vi "Generate_WayPoints_Hopping_LineScan_NOLIGHT.vi"(11 "Input Cluster":T2={"Scan Rate (um/s)"=15.0, "X Start"=15.0, "X End"=15.0, "Y Start"=15.0, "Num_Lines"=15.0, " Z Start"=15.0, "HoppingDistance"=1.0, "V"=15.0, "Z End"=15.0, "Approach Rate Hopping (um/s)"=15.0, "Retract Rate (um/s)"=15.0, "V 2"=15.0, "Approach Rate (um/s)"=15.0}) -> (0 "output cluster":T1)   [LabVIEW 2023]
uses:
  TypeDefs/WayPointCluster.ctl
  User_Vi/Settings.vi
panel:
  out "Numeric":i32
  in  "WayPointCluster":T1
  out "CurrentLine":dbl
  out "X  P":dbl
  out "HoppingDistanceX":dbl
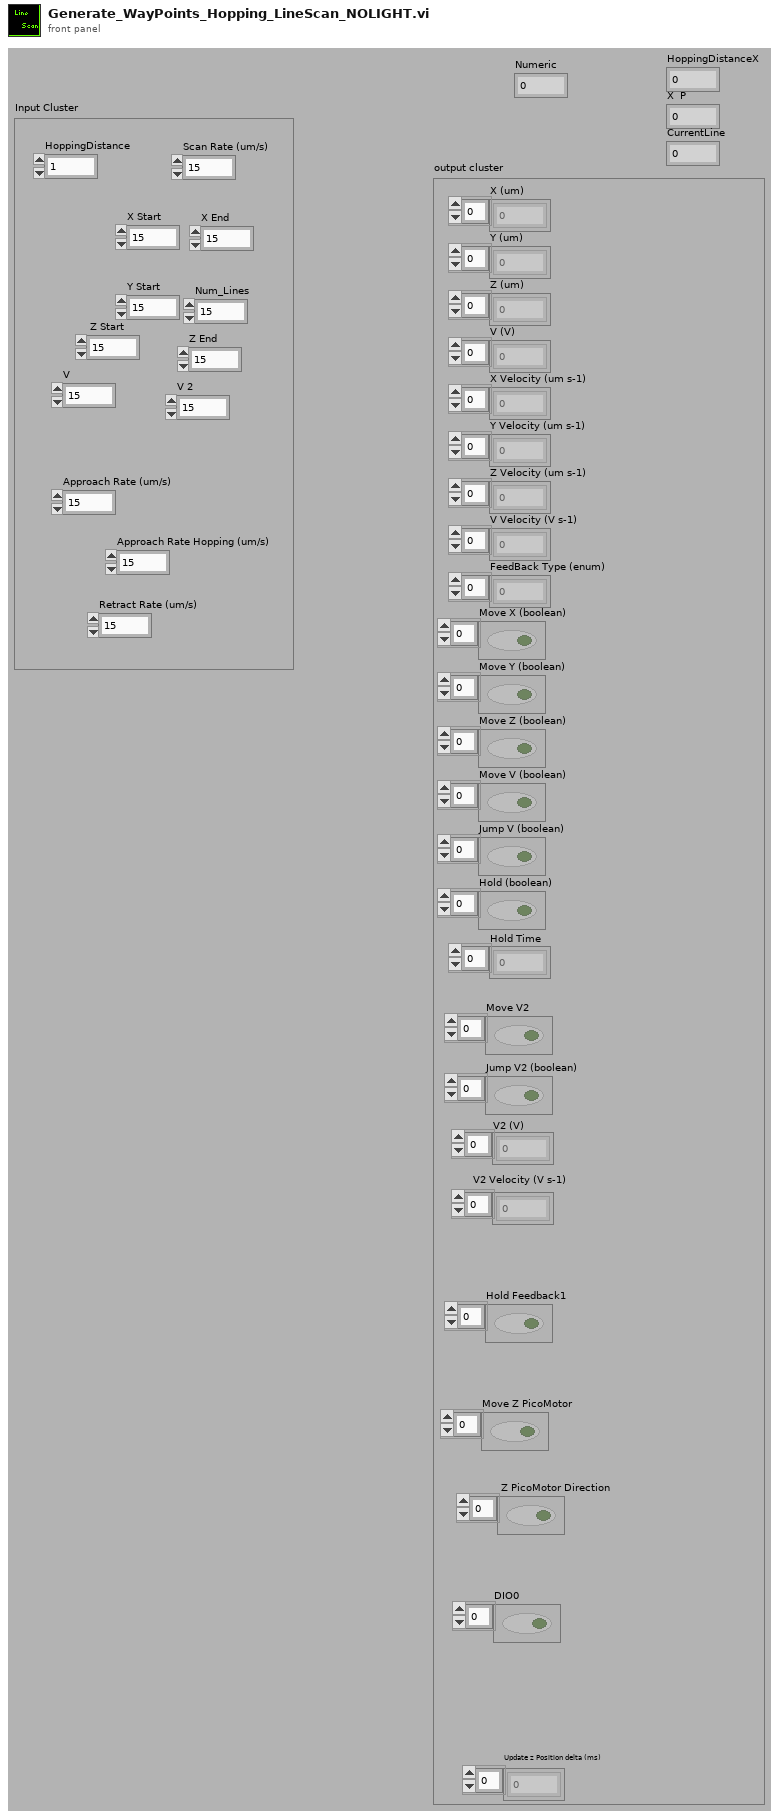
[diagram p1: front panel]
types:
  T1 = typedef "WayPointCluster.ctl" = cluster{"X (um)":dbl[], "Y (um)":dbl[], "Z (um)":dbl[], "V (V)":dbl[], "X Velocity (um s-1)":dbl[], "Y Velocity (um s-1)":dbl[], "Z Velocity (um s-1)":dbl[], "V Velocity (V s-1)":dbl[], "FeedBack Type (enum)":u16[], "Move X (boolean)":bool[], "Move Y (boolean)":bool[], "Move Z (boolean)":bool[], "Move V (boolean)":bool[], "Jump V (boolean)":bool[], "Hold (boolean)":bool[], "Hold Time":u32[], "V2 (V)":dbl[], "Move V2":bool[], "V2 Velocity (V s-1)":dbl[], "Jump V2 (boolean)":bool[], "Update z Position delta (ms)":i16[], "Hold Feedback1":bool[], "Move Z PicoMotor":bool[], " Z PicoMotor Direction":bool[], "DIO0":bool[]}
  T2 = cluster{"Scan Rate (um/s)":dbl, "X Start":dbl, "X End":dbl, "Y Start":dbl, "Num_Lines":dbl, " Z Start":dbl, "HoppingDistance":dbl, "V":dbl, "Z End":dbl, "Approach Rate Hopping (um/s)":dbl, "Retract Rate (um/s)":dbl, "V 2":dbl, "Approach Rate (um/s)":dbl}
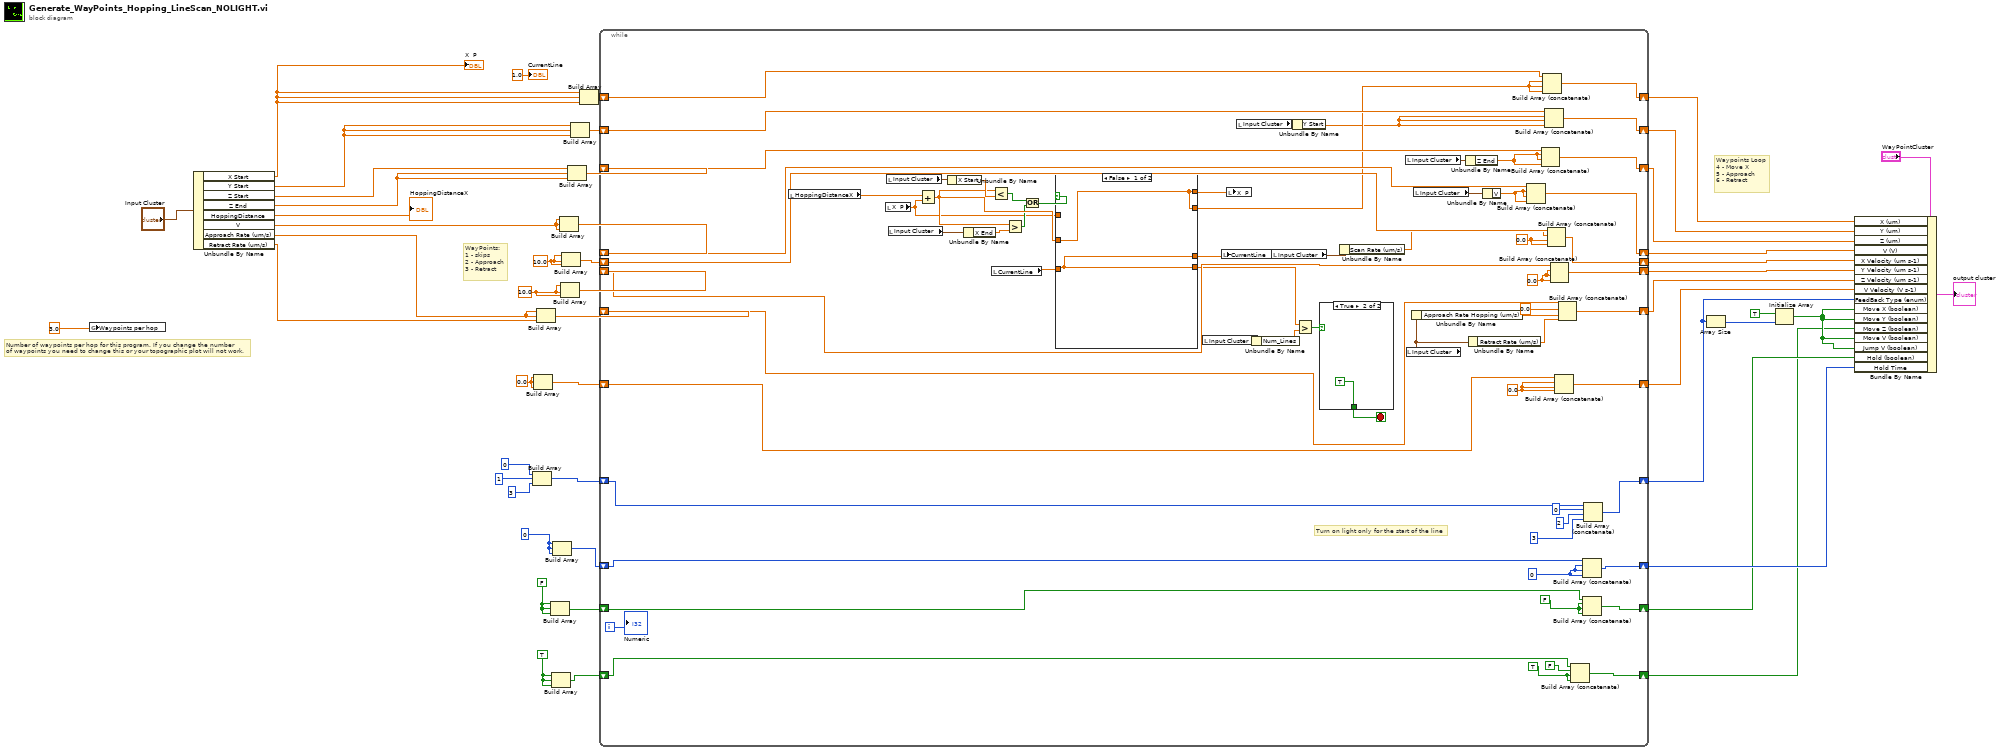
[diagram p0: block diagram]
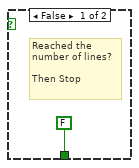
[diagram p2: hidden frame]
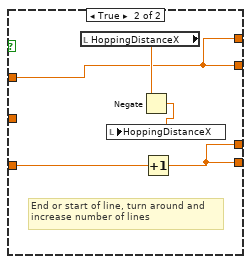
[diagram p3: hidden frame]
diagram:
  w14 = TRUE
  w15 = FALSE
  w23 = u16 0 ("element")
  w9 = 10.0 ("element")
  w10 = 10.0 ("element")
  w12 = 0.0 ("element")
  # "Number of waypoints per hop for this program. If you change the number\nof waypoints you need to change this or your topographic plot will not work."
  # "Waypoints Loop\n4 - Move X\n5 - Approach\n6 - Retract"
  # "WayPoints:\n1 - skips\n2 - Approach\n3 - Retract"
  n1 = global write "Settings.vi" "Waypoints per hop"(3.0) -> ()
  n2 = Unbundle By Name("Input Cluster") -> ("X Start"=w6:dbl, "Y Start"=w5:dbl, "Z Start"=w30:dbl, "Z End"=w7:dbl, "HoppingDistance"=→"HoppingDistanceX":dbl, "V"=w8:dbl, "Approach Rate (um/s)"=w27:dbl, "Retract Rate (um/s)"=w11:dbl)
  "X  P" <- w6
  n3 = Build Array(u16 0 ("element"), u16 1 ("element"), u16 3 ("element")) -> (w33:u16[])
  n4 = Build Array(w12, w12, w12) -> (w24:dbl[])
  n5 = Build Array(w27, w27, w11) -> (w36:dbl[])
  n6 = Build Array(w15, w15, w15) -> (w19:bool[])
  n7 = Build Array(w14, w14, w14) -> (w17:bool[])
  n8 = Build Array(w23, w23, w23) -> (w22:u16[])
  n9 = Build Array(w8, w8, w8) -> (w41:dbl[])
  n10 = Build Array(w10, w10, w10) -> (w38:dbl[])
  n11 = Build Array(w9, w9, w9) -> (w39:dbl[])
  n12 = Build Array(w30, w7, w7) -> (w43:dbl[])
  n13 = Build Array(w5, w5, w5) -> (w44:dbl[])
  n14 = Build Array(w6, w6, w6) -> (w46:dbl[])
  n15 = while {
    shift-right: [w112] -> w45
    shift-left: w46 -> [w113]
    shift-right: [w104] -> w31
    shift-left: w44 -> [w95]
    shift-right: [w103] -> w42
    shift-left: w43 -> [w111]
    shift-right: [w102] -> w40
    shift-left: w41 -> [w110]
    shift-right: [w101] -> w3
    shift-left: w39 -> [w109]
    shift-right: [w77] -> w37
    shift-left: w38 -> [w108]
    shift-right: [w100] -> w35
    shift-left: w36 -> [w107]
    shift-right: [w99] -> w34
    shift-left: w24 -> [w106]
    shift-right: [w98] -> w29
    shift-left: w33 -> [w105]
    shift-right: [w71] -> w21
    shift-left: w22 -> [w72]
    shift-right: [w70] -> w20
    shift-left: w19 -> [w68]
    shift-right: [w65] -> w16
    shift-left: w17 -> [w64]
    i -> [w67]
    stop <- w85 stop-if-true
    w66 = TRUE
    w69 = FALSE
    w62 = u16 0 ("element")
    w59 = 0.0 ("element")
    w58 = 0.0 ("element")
    w61 = 0.0 ("element")
    # "Turn on light only for the start of the line"
    n16 = local read "HoppingDistanceX"() -> (w78:dbl)
    n17 = local read "X  P"() -> (w79:dbl)
    n18 = local read "Input Cluster"() -> (w115:T2)
    n19 = local read "Input Cluster"() -> (w114:T2)
    n20 = Add(x=w78, y=w79) -> (x+y=w91:dbl)
    n21 = Unbundle By Name(w115) -> ("X Start"=w94:dbl)
    n22 = Unbundle By Name(w114) -> ("X End"=w92:dbl)
    n23 = local read "CurrentLine"() -> (w55:dbl)
    n24 = Less?(x=w91, y=w94) -> (x < y?=w93:bool)
    n25 = Greater?(x=w91, y=w92) -> (0:w90:bool)
    n26 = Or(x=w93, y=w90) -> (x .or. y?=w89:bool)
    n27 = case shown="False" w89 {
      tunnel: w91 -> [w119 _]
      tunnel: [w119 w122] -> w56
      tunnel: w79 -> [_ w122]
      tunnel: [w118 w121] -> w84
      tunnel: [w118 w121] -> w83
      tunnel: [w119 w122] -> w63
      tunnel: w55 -> [w118 w120]
      frame False {
      }
      frame True {
        # "End or start of line, turn around and \nincrease number of lines"
        n28 = local read "HoppingDistanceX"() -> (w124:dbl)
        n29 = Negate(x=w124) -> (-x=w123:dbl)
        n30 = local write "HoppingDistanceX"(w123) -> ()
        n31 = Increment(x=w120) -> (x+1=w121:dbl)
      }
    }
    n32 = local read "Input Cluster"() -> (w88:T2)
    n33 = local write "CurrentLine"(w83) -> ()
    n34 = local write "X  P"(w63) -> ()
    n35 = local read "Input Cluster"() -> (w73:T2)
    n36 = Unbundle By Name(w88) -> ("Num_Lines"=w87:dbl)
    n37 = local read "Input Cluster"() -> (w52:T2)
    n38 = Unbundle By Name(w73) -> ("Y Start"=w50:dbl)
    n39 = Greater?(x=w84, y=w87) -> (0:w86:bool)
    n40 = case shown="True" w86 {
      tunnel: [FALSE TRUE] -> w85
      frame False {
        # "Reached the \nnumber of lines?\n\nThen Stop"
      }
      frame True {
      }
    }
    n41 = Unbundle By Name(w52) -> ("Scan Rate (um/s)"=w51:dbl)
    n42 = local read "Input Cluster"() -> (w97:T2)
    n43 = local read "Input Cluster"() -> (w76:T2)
    n44 = Unbundle By Name(w76) -> ("Approach Rate Hopping (um/s)"=w80:dbl)
    n45 = local read "Input Cluster"() -> (w96:T2)
    n46 = Unbundle By Name(w97) -> ("Z End"=w54:dbl)
    n47 = Unbundle By Name(w76) -> ("Retract Rate (um/s)"=w74:dbl)
    n48 = Unbundle By Name(w96) -> ("V"=w57:dbl)
    n49 = Build Array (concatenate)(w110, w57, w57, w57) -> (w102:dbl[])
    n50 = Build Array (concatenate)(w111, w54, w54, w54) -> (w103:dbl[])
    n51 = Build Array (concatenate)(w113, w56, w56, w56) -> (w112:dbl[])
    n52 = Build Array (concatenate)(w95, w50, w50, w50) -> (w104:dbl[])
    n53 = Build Array (concatenate)(w109, w51, w58, w58) -> (w101:dbl[])
    n54 = Build Array (concatenate)(w108, w59, w59, w59) -> (w77:dbl[])
    n55 = Build Array (concatenate)(w106, w61, w61, w61) -> (w99:dbl[])
    n56 = Build Array (concatenate)(w107, 0.0 ("element"), w80, w74) -> (w100:dbl[])
    n57 = Build Array (concatenate)(w64, FALSE, w66, w66) -> (w65:bool[])
    n58 = Build Array (concatenate)(w72, w62, w62, w62) -> (w71:u16[])
    n59 = Build Array (concatenate)(w68, w69, w69, w69) -> (w70:bool[])
    n60 = Build Array (concatenate)(w105, u16 0 ("element"), u16 2 ("element"), u16 3 ("element")) -> (w98:u16[])
    "Numeric" <- w67
  }
  n61 = Array Size(array=w29) -> (size(s)=w32:i32)
  n62 = Initialize Array(TRUE, w32) -> (w18:bool[])
  n63 = Bundle By Name(cluster="WayPointCluster", "X (um)"=w45, "Y (um)"=w31, "Z (um)"=w42, "V (V)"=w40, "X Velocity (um s-1)"=w3, "Y Velocity (um s-1)"=w37, "Z Velocity (um s-1)"=w35, "V Velocity (V s-1)"=w34, "FeedBack Type (enum)"=w29, "Move X (boolean)"=w18, "Move Y (boolean)"=w18, "Move Z (boolean)"=w16, "Move V (boolean)"=w18, "Jump V (boolean)"=w18, "Hold (boolean)"=w20, "Hold Time"=w21) -> (→"output cluster":T1)
  "CurrentLine" <- 1.0 ("Y  P")
